vi "UHR-Fleezers Control (host) -Leonardo 04-2018 V2.vi"(0 "Tab Control":T5(tab)=enum."Trap Control (RF)") -> ()   [LabVIEW 2013] (continued)
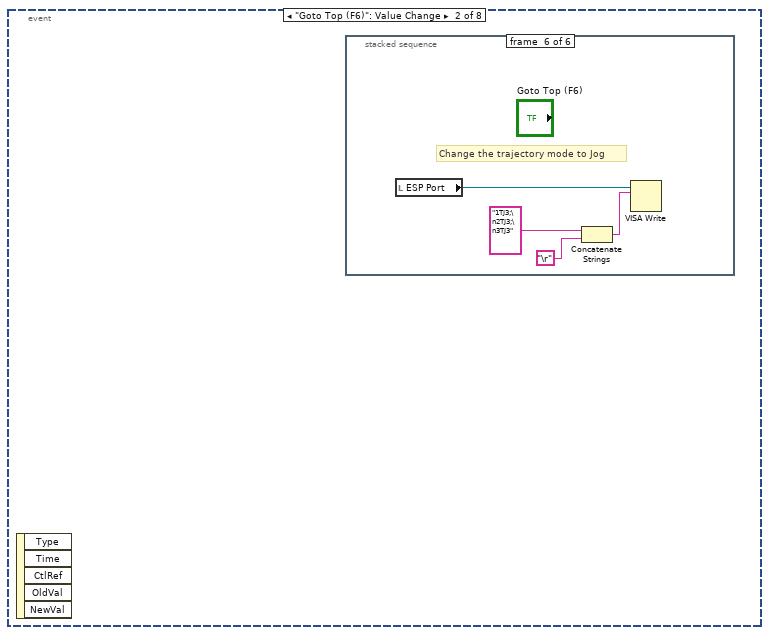
[diagram p4: hidden frame]
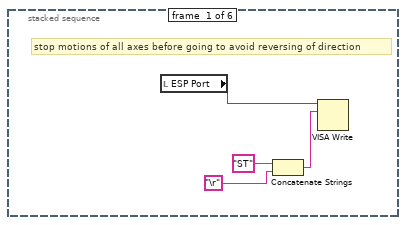
[diagram p5: hidden frame]
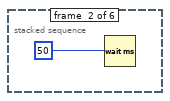
[diagram p6: hidden frame]
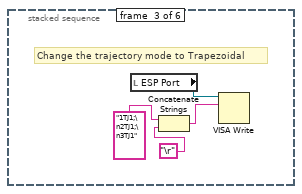
[diagram p7: hidden frame]
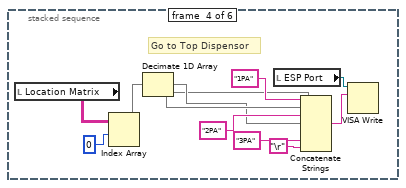
[diagram p8: hidden frame]
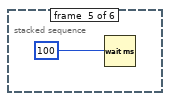
[diagram p9: hidden frame]
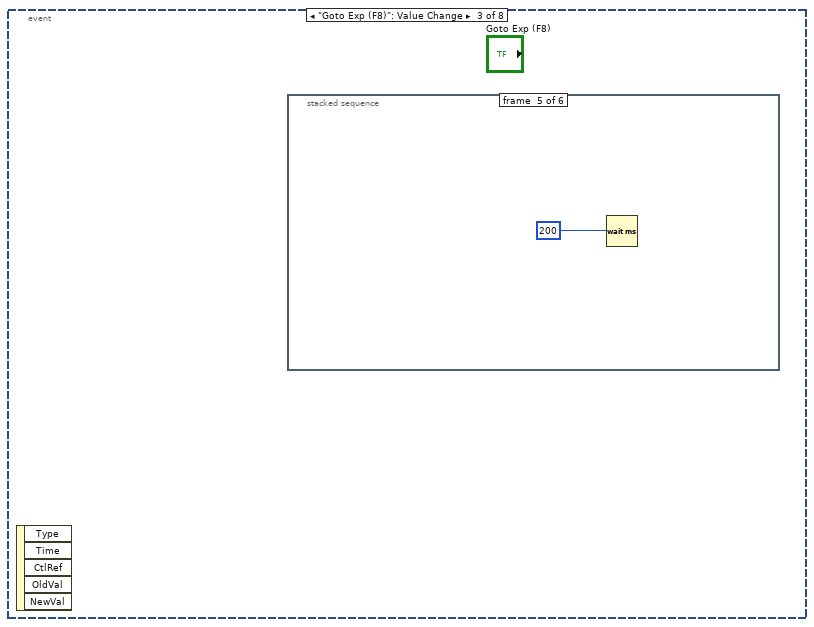
[diagram p10: hidden frame]
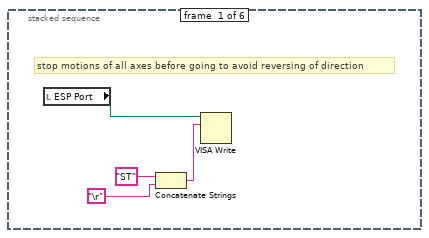
[diagram p11: hidden frame]
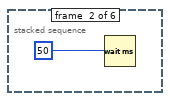
[diagram p12: hidden frame]
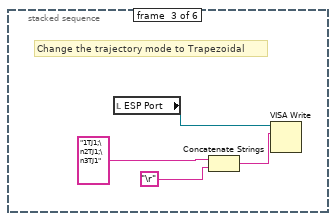
[diagram p13: hidden frame]
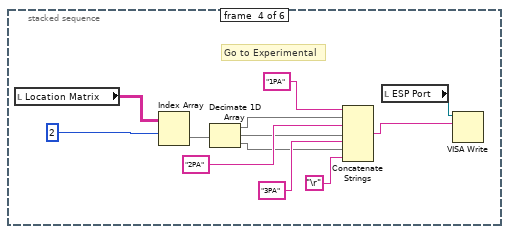
[diagram p14: hidden frame]
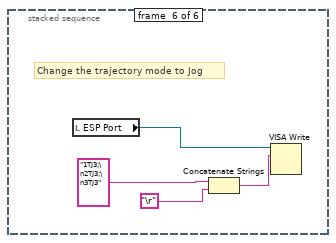
[diagram p15: hidden frame]
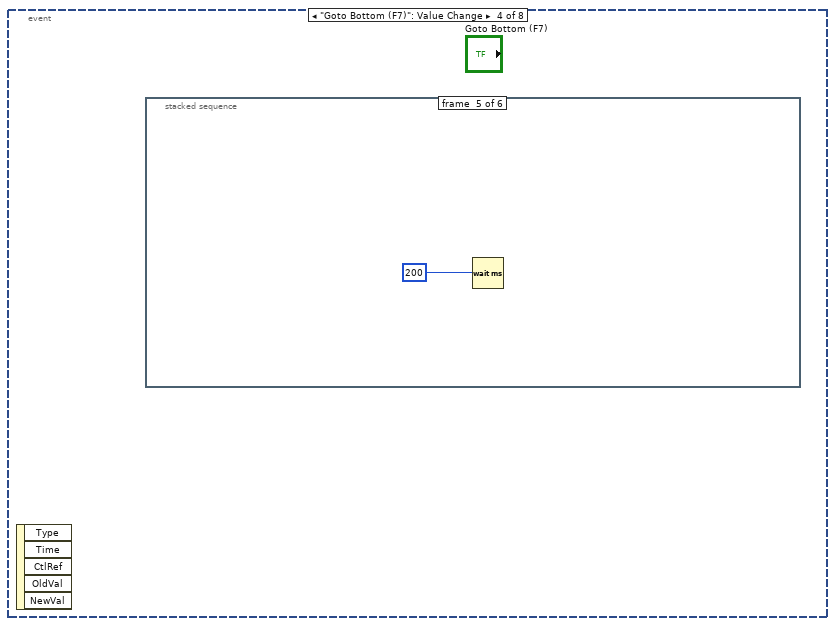
[diagram p16: hidden frame]
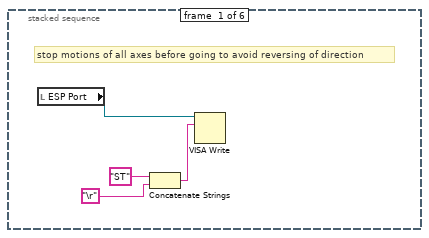
[diagram p17: hidden frame]
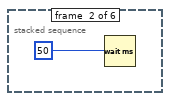
[diagram p18: hidden frame]
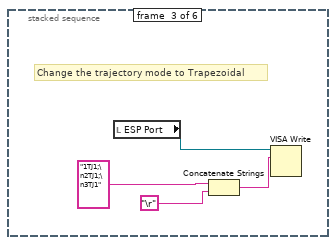
[diagram p19: hidden frame]
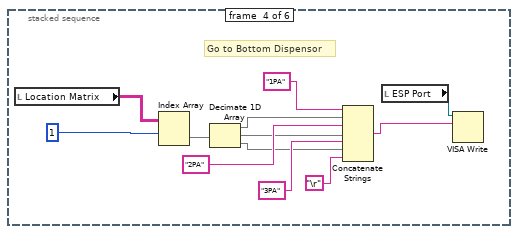
[diagram p20: hidden frame]
    "Green FB Signals (V)" <- w2392
    n2330 = case shown="True" w2147 {
      tunnel: w2146 -> [_ w2497]
      tunnel: w2145 -> [_ w2496]
      frame False {
      }
      frame True {
        w2498 = 50.0
        n2331 = Greater?(x=w2496, y=w2498) -> (0:w2494:bool)
        n2332 = Greater?(x=w2497, y=w2498) -> (0:w2495:bool)
        n2333 = Or(x=w2495, y=w2494) -> (x .or. y?=w2493:bool)
        n2334 = case shown="True" w2493 {
          frame False {
          }
          frame True {
            n2335 = property on="All FB On/Off" class="Bool (strict)"("Val(Sgnl)"=FALSE) -> ()  [unwired: 2 in, 2 out]
            "Feedback overload" <- TRUE
          }
        }
      }
    }
    n2336 = Unbundle By Name(w2392) -> ("Green FB Ch 2"=→"Green FB Plot":dbl)
    n2337 = local read "wait to reset values"() -> (w2476:bool)
    n2338 = Not(x=w2473) -> (.not. x?=w2477:bool)
    n2339 = And(x=w2477, y=w2476) -> (x .and. y?=w2478:bool)
    n2340 = case "Part of MCL raster scanning: returns to initial positions after scan done" shown="True" w2478 {
      tunnel: w2481 -> [w3322 w3329]
      tunnel: [w3322 w3328] -> w2480
      tunnel: w2475 -> [w3321 w3327]
      tunnel: [w3321 w3326] -> w2474
      frame False {
      }
      frame True {
        w3337 = 10.0 ("y")
        w3336 = 32767.0 ("y")
        # "to return scan values\nafter a synchronous \nAOM scan"
        n2341 = local read "AO2"() -> (w3330:dbl)
        n2342 = local read "AO1"() -> (w3331:dbl)
        n2343 = local write "wait to reset values"(FALSE ("wait to reset values")) -> ()
        n2344 = Multiply(x=w3331, y=w3336) -> (x*y=w3333:dbl)
        n2345 = Multiply(x=w3330, y=w3336) -> (x*y=w3335:dbl)
        n2346 = Divide(x=w3333, y=w3337) -> (x/y=w3332:dbl)
        n2347 = Divide(x=w3335, y=w3337) -> (x/y=w3334:dbl)
        n2348 = To Word Integer(number=w3332) -> (16bit integer=w3338:i16)
        n2349 = To Word Integer(number=w3334) -> (16bit integer=w3339:i16)
        n2350 = local read "Total Counts (ticks)"() -> (w3323:u32)
        n2351 = xnode "Read/Write Control"("FPGA VI Reference In"=w3329, "error in"=w3327, "AO1 (Y)"=w3338, "AO2 (X)"=w3339, "MCL count"=w3323) -> ("FPGA VI Reference Out"=w3328:T20, "error out"=w3326:errorcluster)
        n2352 = local read "Scan Range (V)\n(of steps)"() -> (w3324:dbl)
        n2353 = property on="Scan Range (V)\n(of steps)" class="DigNum (strict)"("Val(Sgnl)"=w3324) -> ()  [unwired: 2 in, 2 out]
      }
    }
    n2354 = node-c288() -> ()  [unwired: 2 out]
  }
  n2355 = node-c288(3 ("Processor")) -> (w102:T25)  [unwired: 3 out]
  n2356 = timed-loop "Oscillate AOD (debugging)" {
    tunnel: w55 -> [w3901]
    tunnel: [w3900] -> w66
    timing: w102 -> [_]
    timing-out: [_] -> w101
    stop <- w3900 stop-if-true
    n2357 = node-c288() -> ()  [unwired: 2 out]
    n2358 = event shown="[0] \"Oscillate Set 2\", \"Fish for Tether\": Value Change" {
      selector: _ -> [_ _ _]
      dyn-events: _ -> [_ _ _]
      timeout: _ -> [_ _ _]
      tunnel: w3901 -> [w3908 _ _]
      tunnel: [FALSE ("Stop All") _ w4176] -> w3900
      event "Oscillate Set 2", "Fish for Tether": Value Change {
        n2359 = event-data() -> ()  [unwired: 6 out]
        n2360 = local read "Oscillate Set 2"() -> (w3907:bool)
        n2361 = Or(x=w3907, y="Fish for Tether") -> (x .or. y?=w3905:bool)
        n2362 = case shown="True" w3905 {
          tunnel: w3908 -> [_ w3911]
          tunnel: "Fish for Tether" -> [_ w3910]
          frame False {
          }
          frame True {
            n2363 = case shown="True" w3910 {
              frame False {
              }
              frame True {
                n2364 = local write "Scan axis 2"(TRUE) -> ()
                n2365 = local write "Tether"(FALSE ("Tether")) -> ()
              }
            }
            n2366 = node-c288("Period") -> (w3913:T25)  [unwired: 3 out]
            n2367 = timed-loop "Oscillate AOD" {
              timing: w3913 -> [_]
              timing-out: [_] -> w3912
              tunnel: w3911 -> [w3923]
              tunnel: w3910 -> [w3922]
              i -> [w3925]
              stop <- w3921 stop-if-true
              n2368 = node-c288() -> (w3924:i64)  [unwired: 1 out]
              n2369 = flat-sequence {
                tunnel: w3925 -> [w3951]
                tunnel: w3924 -> [w3950]
                tunnel: w3923 -> [w3934]
                tunnel: w3922 -> [w3936]
                tunnel: [w3936] -> w3920
                tunnel: [w3935] -> w3919
                tunnel: [w3933] -> w3918
                tunnel: [w3930] -> w3916
                tunnel: w3920 -> [w3987]
                tunnel: w3919 -> [w3985]
                tunnel: w3918 -> [w3984]
                tunnel: [w3983] -> w3917
                tunnel: w3916 -> [w3982]
                tunnel: [w4051] -> w3921
                tunnel: w3917 -> [w4049]
                frame #0 {
                  n2370 = Divide(x=w3950, y=i64 1000) -> (x/y=w3945:dbl)
                  n2371 = Multiply(x=w3945, y=w3951) -> (x*y=w3947:dbl)
                  n2372 = Multiply(x="Osc. freq. (Hz)", y=6.283185307179586) -> (x*y=w3948:dbl)
                  n2373 = Multiply(x=w3948, y=w3947) -> (x*y=w3932:dbl)
                  n2374 = local read "BD 1 Frequency 2 (MHz)"() -> (w3929:dbl)
                  n2375 = local read "BD 1 Frequency 1 (MHz)"() -> (w3926:dbl)
                  n2376 = case shown="True" w3936 {
                    tunnel: w3932 -> [w3957 w3964]
                    tunnel: w3929 -> [_ w3974]
                    tunnel: [w3954 w3958] -> w3937
                    tunnel: [FALSE w3967] -> w3933
                    tunnel: [0.0 w3960] -> w3930
                    tunnel: w3926 -> [_ w3959]
                    frame False {
                      n2377 = Sine(x=w3957) -> (sin(x)=w3955:dbl)
                      n2378 = Multiply(x=w3955, y="Osc. amp. (MHz)") -> (x*y=w3954:dbl)
                    }
                    frame True {
                      n2379 = Cosine(x=w3964) -> (cos(x)=w3977:dbl)
                      n2380 = Subtract(x=w3974, y=w3959) -> (x-y=w3973:dbl)
                      n2381 = Decrement(x=w3977) -> (x-1=w3976:dbl)
                      n2382 = Subtract(x=w3973, y="Closest Delta (MHz)") -> (x-y=w3970:dbl)
                      n2383 = Divide(x=w3976, y=2.0) -> (x/y=w3971:dbl)
                      n2384 = Multiply(x=w3971, y=w3970) -> (x*y=w3958:dbl)
                      n2385 = local read "Vec Mean of T1 T2"() -> (w3966:dbl[])
                      n2386 = Greater?(x=w3966, y="Stop F (pN)") -> (0:w3968:bool[])
                      n2387 = Or Array Elements(Boolean array=w3968) -> (logical OR=w3967:bool)
                      n2388 = Divide(x=w3964, y=6.283185307179586) -> (x/y=w3963:dbl)
                      n2389 = Round Toward +Infinity(x=w3963) -> (ceil(x): smallest int >= x=w3960:dbl)
                      "Attempts" <- w3960
                      n2390 = Greater?(x=w3960, y="Attempt Limit") -> (0:w3962:bool)
                      n2391 = case shown="True" w3962 {
                        frame False {
                        }
                        frame True {
                          n2392 = local write "Fish for Tether"(FALSE ("Fish for Tether")) -> ()
                          n2393 = call <vilib>:"Beep.vi"() -> ()  [unwired: 3 in, 9 out]
                          n2394 = local read "Messages"() -> (w3979:string)
                          n2395 = call "Update messages.vi"("Message to add"="Tether fishing timeout." ("Messages"), "Old message string"=w3979) -> ("New message string"=→"Messages":string)
                        }
                      }
                    }
                  }
                  n2396 = local read "Y RF Frequency Limits (MHz)"() -> (w3938:T16)
                  n2397 = local read "X RF Frequency Limits (MHz)"() -> (w3939:T16)
                  n2398 = local read "BD 1 Frequency 3 (MHz)"() -> (w3944:dbl)
                  n2399 = local read "BD 2 Frequency 2 (MHz)"() -> (w3928:dbl)
                  n2400 = Select(t=w3929, s="Scan axis 2", f=w3928) -> (s? t:f=w3940:dbl)
                  n2401 = Add(x=w3937, y=w3940) -> (x+y=w3935:dbl)
                  n2402 = Select(t=w3935, s="Scan axis 2", f=w3929) -> (s? t:f=w3927:dbl)
                  n2403 = Select(t=w3928, s="Scan axis 2", f=w3935) -> (s? t:f=w3942:dbl)
                  n2404 = local read "BD 2 Frequency 3 (MHz)"() -> (w3943:dbl)
                  n2405 = call "set RF board frequency - interlace.vi"("Board 2 Frequency Limits"=w3938, "Board 1 Frequency Limits"=w3939, "FPGA VI Reference In"=w3934, "Board 2 Frequency 3 (MHz)"=w3943, "Board 1 Frequency 3 (MHz)"=w3944, "Board 2 Frequency 2 (MHz)"=w3928, "Board 2 Frequency 1 (MHz)"=w3942, "Board 1 Frequency 2 (MHz)"=w3927, "Board 1 Frequency 1  (MHz)"=w3926) -> ()  [unwired: 1 in, 2 out]
                }
                frame #1 {
                  n2406 = And(x=w3987, y=w3984) -> (x .and. y?=w3986:bool)
                  n2407 = case "Only if were fishing and now formed tether" shown="True" w3986 {
                    tunnel: w3985 -> [w3989 w4001]
                    tunnel: [w3988 w4000] -> w3983
                    tunnel: w3982 -> [_ w3996]
                    frame False {
                      n2408 = local read "Fish for Tether"() -> (w3988:bool)
                      n2409 = case shown="True" w3988 {
                        tunnel: w3989 -> [_ _]
                        frame False {
                        }
                        frame True {
                        }
                      }
                    }
                    frame True {
                      w4000 = FALSE ("Fish for Tether")
                      n2410 = call <vilib>:"Beep.vi"() -> ()  [unwired: 3 in, 9 out]
                      n2411 = Number To Decimal String(number=w3996, width (-)=i16 1) -> (decimal integer string=w3994:string)
                      n2412 = case shown="\"2\", \"3\", \"4\", \"5\", \"6\"" "Then..." {
                        selector: "Then..." -> [_ w4004]
                        tunnel: w4001 -> [w4003 _]
                        frame "1", Default {
                          # "do nothing"
                          n2413 = property on="BD 1 Frequency 1 (MHz)" class="DigNum (strict)"("Val(Sgnl)"=w4003) -> ()  [unwired: 2 in, 2 out]
                        }
                        frame "2", "3", "4", "5", "6" {
                          n2414 = flat-sequence {
                            tunnel: w4004 -> [w4006]
                            frame #0 {
                              n2415 = property on="Trap Delta (MHz)" class="DigNum (strict)"("Val(Sgnl)"="Move to Delta 1 (MHz)") -> ()  [unwired: 2 in, 2 out]
                            }
                            frame #1 {
                              n2416 = case shown="\"5\", \"6\"" w4006 {
                                selector: w4006 -> [w4009 w4019 _]
                                frame "3", "4" {
                                n2417 = flat-sequence {
                                tunnel: w4009 -> [w4010]
                                tunnel: [w4010] -> w4007
                                tunnel: [w4012] -> w4008
                                tunnel: w4007 -> [w4012]
                                tunnel: w4008 -> [w4016]
                                frame #0 {
                                n2418 = property on="Green Laser ON/Interlacing" class="Bool (strict)"("Val(Sgnl)"=TRUE ("Value (Signaling)")) -> ()  [unwired: 2 in, 2 out]
                                }
                                frame #1 {
                                n2419 = Multiply(x="Wait Before Save (s)", y=u32 1000 ("x")) -> (x*y=w4014:u32)
                                n2420 = Wait (ms)(milliseconds to wait=w4014) -> ()  [unwired: 1 out]
                                }
                                frame #2 {
                                n2421 = property on="Start Saving" class="Bool (strict)"("Value"=TRUE ("Start Saving")) -> ()  [unwired: 2 in, 2 out]
                                n2422 = case shown="Default" w4016 {
                                frame Default {
                                }
                                frame "4" {
                                n2423 = property on="Fl. Triggered..." class="Bool (strict)"("Val(Sgnl)"=TRUE ("Value (Signaling)")) -> ()  [unwired: 2 in, 2 out]
                                }
                                }
                                }
                                }
                                }
                                frame "5", "6" {
                                n2424 = stacked-sequence {
                                tunnel: w4019 -> [_ _ _ _ _ _ _ _ w4036 _ _]
                                frame #0 {
                                n2425 = Replace Array Subset(array=u32[] [0] ("Index Values"), new element="Raster Set Upon Tether", index=0) -> (w4020:u32[])
                                n2426 = property on="Saved AOD Raster Scan Parameter Sets" class="Arr (strict)"("Index Values"=w4020) -> ()  [unwired: 2 in, 2 out]
                                }
                                frame #1 {
                                n2427 = Wait (ms)(milliseconds to wait=u32 500) -> ()  [unwired: 1 out]
                                }
                                frame #2 {
                                n2428 = property on="Load parameters" class="Bool (strict)"("Val(Sgnl)"=TRUE ("Value (Signaling)")) -> ()  [unwired: 2 in, 2 out]
                                }
                                frame #3 {
                                n2429 = Wait (ms)(milliseconds to wait=u32 500) -> ()  [unwired: 1 out]
                                }
                                frame #4 {
                                n2430 = property on="Trap Raster Scan" class="Bool (strict)"("Val(Sgnl)"=TRUE ("Value (Signaling)")) -> ()  [unwired: 2 in, 2 out]
                                }
                                frame #5 {
                                n2431 = Wait (ms)(milliseconds to wait=u32 2000) -> ()  [unwired: 1 out]
                                }
                                frame #6 {
                                n2432 = while {
                                stop <- w4031 stop-if-true
                                n2433 = local read "Raster Scanning..."() -> (w4030:bool)
                                n2434 = local read "Saving..."() -> (w4033:bool)
                                n2435 = Wait (ms)(milliseconds to wait=u32 100) -> ()  [unwired: 1 out]
                                n2436 = Not(x=w4033) -> (.not. x?=w4032:bool)
                                n2437 = Not(x=w4030) -> (.not. x?=w4029:bool)
                                n2438 = And(x=w4032, y=w4029) -> (x .and. y?=w4031:bool)
                                }
                                }
                                frame #7 {
                                n2439 = property on="Trap Delta (MHz)" class="DigNum (strict)"("Val(Sgnl)"="Move to Delta 2 (MHz)") -> ()  [unwired: 2 in, 2 out]
                                }
                                frame #8 {
                                n2440 = local read "Tether"() -> (w4037:bool)
                                n2441 = case shown="True" w4037 {
                                tunnel: w4036 -> [_ w4038]
                                frame False {
                                }
                                frame True {
                                n2442 = flat-sequence {
                                tunnel: w4038 -> [w4040]
                                frame #0 {
                                n2443 = Wait (ms)(milliseconds to wait=u32 500) -> ()  [unwired: 1 out]
                                }
                                frame #1 {
                                n2444 = case shown="\"6\"" w4040 {
                                frame Default {
                                }
                                frame "6" {
                                n2445 = property on="Green Laser ON/Interlacing" class="Bool (strict)"("Val(Sgnl)"=TRUE ("Green Laser ON/Interlacing")) -> ()  [unwired: 2 in, 2 out]
                                }
                                }
                                }
                                frame #2 {
                                n2446 = Wait (ms)(milliseconds to wait=u32 500) -> ()  [unwired: 1 out]
                                }
                                frame #3 {
                                n2447 = local write "Start Saving"("Save at end (5, 6)") -> ()
                                }
                                }
                                }
                                }
                                }
                                frame #9 {
                                n2448 = local read "Bead Sep. Int. Time (s)"() -> (w4046:dbl)
                                n2449 = Multiply(x=w4046, y=1000.0) -> (x*y=w4045:dbl)
                                n2450 = Wait (ms)(milliseconds to wait=w4045) -> ()  [unwired: 1 out]
                                }
                                frame #10 {
                                n2451 = property on="Rescale on Mean" class="Bool (strict)"("Val(Sgnl)"=TRUE ("Value (Signaling)")) -> ()  [unwired: 2 in, 2 out]
                                }
                                }
                                }
                                frame "2", Default {
                                }
                              }
                            }
                          }
                        }
                      }
                      n2452 = Concatenate Strings("Formed tether in ", w3994, " attempt(s)." ("string")) -> (w3991:string)
                      n2453 = local read "Messages"() -> (w3998:string)
                      n2454 = local write "Fish for Tether"(w4000) -> ()
                      n2455 = call "Update messages.vi"("Message to add"=w3991, "Old message string"=w3998) -> ("New message string"=w3997:string)
                      n2456 = local write "Messages"(w3997) -> ()
                      n2457 = Get Date/Time In Seconds() -> (seconds since 1Jan1904=→"Time tether formed":timestamp)
                      "Tether" <- "Tether Alarm?"
                    }
                  }
                }
                frame #2 {
                  n2458 = local read "Oscillate Set 2"() -> (w4050:bool)
                  n2459 = local read "Stop All"() -> (w4052:bool)
                  n2460 = Not Or(1:w4049, 2:w4050) -> (0:w4048:bool)
                  n2461 = Compound Arithmetic op=OR(w4052, w4048) -> (w4051:bool)
                }
              }
              n2462 = node-c288() -> ()  [unwired: 2 out]
            }
            n2463 = node-c288(w3912) -> ()  [unwired: 1 out]
          }
        }
      }
      event "Fl. Triggered...": Value Change {
        n2464 = event-data() -> ()  [unwired: 7 out]
        n2465 = case shown="True" "Fl. Triggered..." {
          frame False {
          }
          frame True {
            n2466 = node-c288() -> (w4064:T25)  [unwired: 4 out]
            n2467 = timed-loop {
              timing: w4064 -> [_]
              timing-out: [_] -> w4063
              tunnel: "Action" -> [w4068]
              shift-right: [w4065] -> _
              shift-left: u8 255 -> [w4067]
              stop <- w4069 stop-if-true
              n2468 = node-c288() -> ()  [unwired: 2 out]
              n2469 = flat-sequence {
                tunnel: w4068 -> [w4081]
                tunnel: w4067 -> [w4078]
                tunnel: [w4077] -> w4066
                tunnel: [w4167] -> w4069
                tunnel: w4066 -> [w4166]
                tunnel: [w4166] -> w4065
                frame #0 {
                  n2470 = local read "Delta Fl. 2"() -> (w4072:dbl)
                  n2471 = local read "Delta Fl. 1"() -> (w4073:dbl)
                  n2472 = Select(t=w4073, s="APD to Watch", f=w4072) -> (s? t:f=w4071:dbl)
                  n2473 = Multiply(x="Fl. Delta Thresh. (kHz)", y=1000.0) -> (x*y=w4080:dbl)
                  n2474 = Greater?(x=w4071, y=w4080) -> (0:w4075:bool)
                  n2475 = Or(x="Force Yank", y=w4075) -> (x .or. y?=w4076:bool)
                  n2476 = case shown="True" w4076 {
                    tunnel: w4081 -> [_ w4091]
                    tunnel: w4078 -> [w4083 w4087]
                    tunnel: [w4083 w4084] -> w4077
                    frame False {
                    }
                    frame True {
                      n2477 = flat-sequence {
                        tunnel: w4088 -> [w4097]
                        tunnel: [w4097] -> w4092
                        tunnel: w4091 -> [w4096]
                        tunnel: [w4096] -> w4090
                        tunnel: [w4095] -> w4089
                        tunnel: w4087 -> [w4094]
                        tunnel: [w4093] -> w4086
                        tunnel: w4092 -> [w4122]
                        tunnel: w4090 -> [w4121]
                        tunnel: w4089 -> [w4120]
                        tunnel: w4086 -> [w4119]
                        tunnel: [w4119] -> w4085
                        tunnel: w4085 -> [w4164]
                        tunnel: [w4164] -> w4084
                        frame #0 {
                          n2478 = call <vilib>:"Beep.vi"() -> ()  [unwired: 3 in, 9 out]
                          n2479 = local write "Waiting"(FALSE ("Waiting")) -> ()
                          n2480 = Increment(x=w4094) -> (x+1=w4093:u8)
                          n2481 = case shown="\"Yank\"" w4096 {
                            tunnel: w4093 -> [_ _ w4103]
                            frame "Image" {
                              n2482 = property on="Confocal Image" class="Bool (strict)"("Val(Sgnl)"=TRUE ("Value (Signaling)")) -> ()  [unwired: 2 in, 2 out]
                            }
                            frame "Alarm", Default {
                            }
                            frame "Yank" {
                              n2483 = flat-sequence {
                                tunnel: w4103 -> [w4106]
                                tunnel: [w4105] -> w4102
                                tunnel: ["N Array El"] -> w4101
                                tunnel: w4102 -> [w4116]
                                tunnel: w4101 -> [w4112]
                                frame #0 {
                                n2484 = Multiply(x="Yank Delay (s)", y=1000.0) -> (x*y=w4109:dbl)
                                n2485 = Quotient & Remainder(x=w4106, y="N Array El") -> (x-y*floor(x/y)=w4105:u8)  [unwired: 1 out]
                                n2486 = Wait (ms)(milliseconds to wait=w4109) -> ()  [unwired: 1 out]
                                }
                                frame #1 {
                                n2487 = Random Number (0-1)() -> (number: 0 to 1=w4113:dbl)
                                n2488 = Multiply(x=w4112, y=w4113) -> (x*y=w4111:dbl)
                                n2489 = Round Toward -Infinity(1:w4111) -> (0:w4110:dbl)
                                n2490 = Select(t=w4110, s="Random Choice", f=w4116) -> (s? t:f=w4114:dbl)
                                n2491 = Index Array(array="Yank to Delta Array (MHz)", index=w4114) -> (element=w4117:dbl)
                                n2492 = property on="Trap Delta (MHz)" class="DigNum (strict)"("Val(Sgnl)"=w4117) -> ()  [unwired: 2 in, 2 out]
                                }
                              }
                            }
                          }
                          n2493 = local read "Time (s)"() -> (w4095:dbl)
                          "Fl. High" <- TRUE ("Yanking")
                        }
                        frame #1 {
                          n2494 = node-c288() -> (w4124:T25)  [unwired: 4 out]
                          n2495 = timed-loop {
                            timing: w4124 -> [_]
                            timing-out: [_] -> w4123
                            tunnel: w4122 -> [w4140]
                            tunnel: w4121 -> [w4138]
                            tunnel: w4120 -> [w4137]
                            stop <- w4139 stop-if-true
                            n2496 = node-c288() -> ()  [unwired: 2 out]
                            n2497 = local read "Fl. Delta Thresh. (kHz)"() -> (w4132:dbl)
                            n2498 = local read "Fl. Triggered..."() -> (w4141:bool)
                            n2499 = local read "Delta Fl. 1"() -> (w4128:dbl)
                            n2500 = local read "Delta Fl. 2"() -> (w4126:dbl)
                            n2501 = local read "Stop All"() -> (w4135:bool)
                            n2502 = local read "APD to Watch"() -> (w4127:bool)
                            n2503 = Select(t=w4128, s=w4127, f=w4126) -> (s? t:f=w4125:dbl)
                            n2504 = Not(x=w4141) -> (.not. x?=w4136:bool)
                            n2505 = Multiply(x=w4132, y=1000.0) -> (x*y=w4131:dbl)
                            n2506 = Negate(x=w4131) -> (-x=w4130:dbl)
                            n2507 = Less?(x=w4125, y=w4130) -> (x < y?=w4134:bool)
                            n2508 = Compound Arithmetic op=OR(w4134, w4135, w4136, "Force Reset") -> (w4139:bool)
                            n2509 = case shown="True" w4139 {
                              tunnel: w4140 -> [_ w4152]
                              tunnel: w4138 -> [_ w4151]
                              tunnel: w4137 -> [_ w4149]
                              frame False {
                              }
                              frame True {
                                n2510 = case shown="\"Yank\"" w4151 {
                                tunnel: w4152 -> [_ w4153]
                                frame "Image", Default {
                                }
                                frame "Yank" {
                                n2511 = flat-sequence {
                                tunnel: [w4158] -> w4154
                                tunnel: w4153 -> [w4158]
                                tunnel: w4154 -> [w4159]
                                frame #0 {
                                n2512 = local read "Yank Delay (s)"() -> (w4157:dbl)
                                n2513 = Multiply(x=w4157, y=1000.0) -> (x*y=w4155:dbl)
                                n2514 = Wait (ms)(milliseconds to wait=w4155) -> ()  [unwired: 1 out]
                                }
                                frame #1 {
                                n2515 = property on="Trap Delta (MHz)" class="DigNum (strict)"("Val(Sgnl)"=w4159) -> ()  [unwired: 2 in, 2 out]
                                }
                                }
                                }
                                }
                                n2516 = local read "Time (s)"() -> (w4150:dbl)
                                n2517 = Subtract(x=w4150, y=w4149) -> (x-y=w4146:dbl)
                                "Duration (s)" <- w4146
                                n2518 = Number To Decimal String(number=w4146, width (-)=i16 0) -> (decimal integer string=w4144:string)
                                n2519 = Concatenate Strings(w4144, " s fluorescence event." ("string")) -> (w4142:string)
                                n2520 = local read "Messages"() -> (w4148:string)
                                n2521 = call "Update messages.vi"("Message to add"=w4142, "Old message string"=w4148) -> ("New message string"=w4147:string)
                                n2522 = call <vilib>:"Beep.vi"() -> ()  [unwired: 3 in, 9 out]
                                n2523 = local write "Messages"(w4147) -> ()
                              }
                            }
                            n2524 = node-c288() -> ()  [unwired: 2 out]
                          }
                          n2525 = node-c288(w4123) -> ()  [unwired: 1 out]
                        }
                        frame #2 {
                          n2526 = local write "Fl. High"(FALSE ("Yanking")) -> ()
                        }
                      }
                      n2527 = local read "Trap Delta (MHz)"() -> (w4088:dbl)
                    }
                  }
                }
                frame #1 {
                  n2528 = local read "Stop All"() -> (w4170:bool)
                  n2529 = local read "Fl. Triggered..."() -> (w4168:bool)
                  n2530 = Not(x=w4168) -> (.not. x?=w4169:bool)
                  n2531 = Or(x=w4169, y=w4170) -> (x .or. y?=w4167:bool)
                  n2532 = Not(x=w4167) -> (.not. x?=→"Waiting":bool)
                }
              }
              n2533 = node-c288() -> ()  [unwired: 2 out]
            }
            n2534 = node-c288(w4063) -> ()  [unwired: 1 out]
          }
        }
      }
      event "Stop All": Value Change {
        n2535 = event-data() -> ()  [unwired: 7 out]
        n2536 = local read "Stop All"() -> (w4176:bool)
      }
    }
    n2537 = node-c288() -> ()  [unwired: 2 out]
  }
  n2538 = node-c288(w101) -> ()  [unwired: 1 out]
  n2539 = node-c288(w187) -> ()  [unwired: 1 out]
  n2540 = flat-sequence {
    tunnel: w63 -> [w4181]
    tunnel: [w4180] -> w69
    tunnel: [w4177] -> w68
    tunnel: w67 -> [_]
    tunnel: w66 -> [_]
    tunnel: w65 -> [_]
    tunnel: w64 -> [_]
    tunnel: w62 -> [w4178]
    tunnel: w69 -> [w4184]
    tunnel: w68 -> [w4183]
    frame #0 {
      w4179 = FALSE ("APD to FIFO")
      n2541 = xnode "Read/Write Control"("FPGA VI Reference In"=w4181, "error in"=w4178, "APD to FIFO"=w4179, "AI to FIFO"=w4179) -> ("FPGA VI Reference Out"=w4180:T20, "error out"=w4177:errorcluster)
    }
    frame #1 {
      n2542 = xnode "Invoke Method"("FPGA VI Reference In"=w4184, "error in"=w4183) -> ("FPGA VI Reference Out"=w4182:T20)  [unwired: 1 out]
      n2543 = xnode "Close FPGA VI Reference"("FPGA VI Reference In"=w4182) -> ()  [unwired: 1 in, 1 out]
    }
  }
